vi "Queue_Driver.vi"   [LabVIEW 2023]
doc: "This is a polymorphic vi that is used to use all the queue driver in single node"
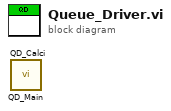
[diagram p0: block diagram]
diagram:
  n1 = call "QD_Main.vi"() -> ()  [unwired: 13 in, 3 out]
  n2 = call "QD_Calci.vi"() -> ()  [unwired: 13 in, 3 out]
